vi "PH_PSDBWriter.PC get Inst ID.vi"(0 "VI in":refnum<vi>, 5 "error in (no error)":errorcluster) -> (14 "VI out":refnum<vi>, 19 "error out":errorcluster)   [LabVIEW 2014, in "PH_PSDBWriter.lvlib"]
uses:
  PH_PSDBWriter.lvlib
  PH_PSDBWriter.Data Status.ctl
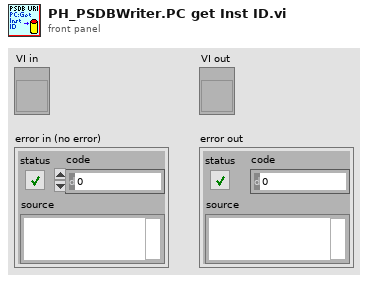
[diagram p1: front panel]
types:
  T1 = typedef "PH_PSDBWriter.lvlib/PH_PSDBWriter.Data Status.ctl" = i16
  T2 = typedef "PH_PSDBWriter.lvlib/PH_PSDBWriter.i attribute.ctl" = cluster{"PSDB Status Service ID":i32, "Instance ID":i32, "Shot #":i32, "Subsystem":T3, "Data Status":T1, "Ref PSDB Status":refnum<vi>, "PSDB Error Code":i32, "PSDB Dataset":T4, "PSDB Thread":cluster{"Ref":refnum<vi>, "Q-Ref":refnum<queue>}, "PSDB Credentials":T12}
  T3 = typedef "PH_PSDBWriter.lvlib/PH_PSDBWriter.PHELIX-Subsystems.ctl" = i32
  T4 = typedef "PH_PSDBWriter.lvlib/PH_PSDBWriter.PSDB Dataset.ctl" = cluster{"Version":i32, "2D data Input":T5[], "Boolean Input":T7[], "Image Input":T8[], "Numeric Input":T10[], "String Input":T11[]}
  T5 = typedef "PH_PSDBWriter.lvlib/PH_PSDBWriter.2D dataset.ctl" = cluster{"name":string, "data":dbl[][], "axis description":T6}
  T6 = typedef "PSDB.lvlib/PSDB_AxisDescription.ctl" = cluster{"x axis label":string, "y axis label":string, "x axis unit":string, "y axis unit":string}
  T7 = typedef "PH_PSDBWriter.lvlib/PH_PSDBWriter.Boolean dataset.ctl" = cluster{"name":string, "data":bool, "unit":string}
  T8 = typedef "PH_PSDBWriter.lvlib/PH_PSDBWriter.Image dataset.ctl" = cluster{"name":string, "data":T9, "unit":string}
  T9 = typedef "IMAQ Image.ctl" = refnum<image>
  T10 = typedef "PH_PSDBWriter.lvlib/PH_PSDBWriter.Numeric dataset.ctl" = cluster{"name":string, "data":dbl, "unit":string}
  T11 = typedef "PH_PSDBWriter.lvlib/PH_PSDBWriter.String dataset.ctl" = cluster{"name":string, "data":string, "unit":string}
  T12 = typedef "PH_Common.lvlib/PH_Connection.PSDB Credentials.ctl" = cluster{"PW":string, "ID":string, "DS":string}
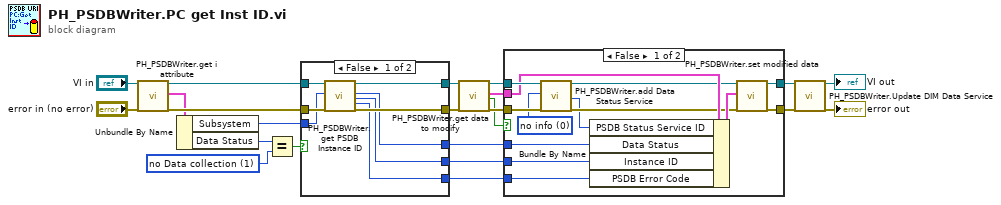
[diagram p0: block diagram]
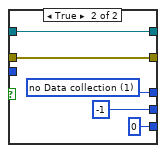
[diagram p2: hidden frame]
diagram:
  w12 = T1 1 items=["no info", "no Data collection", "no problem", "Error getting the instance ID", "Error writing Data to data base"] ("Metadata.Data Status")
  n1 = call "PH_PSDBWriter.get i attribute.vi"("i ref in"="VI in", "error in (no error)"="error in (no error)") -> ("i ref out"=w16:refnum<vi>, "i attribute"=w10:T2, "error out"=w14:errorcluster)  [unwired: 15 in]
  n2 = Unbundle By Name(w10) -> ("Subsystem"=w9:T3, "Data Status"=w11:T1)
  n3 = Equal?(x=w11, y=w12) -> (x = y?=w8:bool)
  n4 = case shown="False" w8 {
    tunnel: w14 -> [w30 w32]
    tunnel: [w24 w35] -> w7
    tunnel: [w25 -1 ("Metadata.Instance ID")] -> w6
    tunnel: w9 -> [w29 _]
    tunnel: w16 -> [w28 w33]
    tunnel: [w27 w32] -> w13
    tunnel: [w26 w33] -> w15
    tunnel: [w23 0 ("PSDB Error Code")] -> w5
    frame False {
      n5 = call "PH_PSDBWriter.get PSDB Instance ID.vi"("i ref in"=w28, "Subsystem"=w29, "error in"=w30) -> ("i ref out"=w26:refnum<vi>, "Metadata.Data Status"=w24:T1, "instance_id"=w25:i32, "PSDB Error Code"=w23:i32, "error out"=w27:errorcluster)  [unwired: 12 in]
    }
    frame True {
      w35 = T1 1 items=["no info", "no Data collection", "no problem", "Error getting the instance ID", "Error writing Data to data base"] ("Metadata.Data Status")
    }
  }
  n6 = call "PH_PSDBWriter.get data to modify.vi"("i ref in"=w15, "error in (no error)"=w13) -> ("i ref out"=w21:refnum<vi>, "i attribute"=w18:T2, "timed out"=w19:bool, "error out"=w20:errorcluster)  [unwired: 14 in]
  n7 = case shown="False" w19 {
    tunnel: w21 -> [w45 w50]
    tunnel: [w47 w50] -> w3
    tunnel: w20 -> [w43 w49]
    tunnel: [w46 w49] -> w1
    tunnel: w18 -> [w44 _]
    tunnel: w7 -> [w38 _]
    tunnel: w6 -> [w37 _]
    tunnel: w5 -> [w36 _]
    frame False {
      w42 = T1 0 items=["no info", "no Data collection", "no problem", "Error getting the instance ID", "Error writing Data to data base", "Error concerning the subsystem", "Error getting the Shot ID", "Error getting the Shot Types", "Error getting the Experiments", "Error verifying wanted Shottype", "Error verifying wanted Experiment"] ("Data Status")
      n8 = call "PH_PSDBWriter.add Data Status Service.vi"("i ref in"=w45, "Data Status"=w42, "error in (no error)"=w43) -> ("i ref out"=w40:refnum<vi>, "Service ID Data Status"=w39:i32, "error out"=w41:errorcluster)  [unwired: 14 in]
      n9 = Bundle By Name(cluster=w44, "PSDB Status Service ID"=w39, "Data Status"=w38, "Instance ID"=w37, "PSDB Error Code"=w36) -> (w48:T2)
      n10 = call "PH_PSDBWriter.set modified data.vi"("i ref in"=w40, "i attribute"=w48, "error in (no error)"=w41) -> ("i ref out"=w47:refnum<vi>, "error out"=w46:errorcluster)  [unwired: 15 in]
    }
    frame True {
    }
  }
  n11 = call "PH_PSDBWriter.Update DIM Data Service.vi"("i ref in"=w3, "error in"=w1) -> ("i ref out"=→"VI out":refnum<vi>, "error out"=→"error out":errorcluster)  [unwired: 16 in]
